vi "CaseNames To CSM States.vi"(11 "Array in":string[](array[string])) -> (3 "Array out":string[](array[string]))   [LabVIEW 2017, in "CSM-Helper.lvclass"]
uses:
  CSM-Helper.lvclass
  _Shared/CSM Shared.lvlib
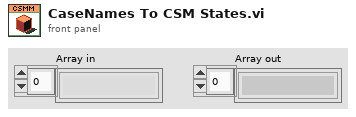
[diagram p1: front panel]
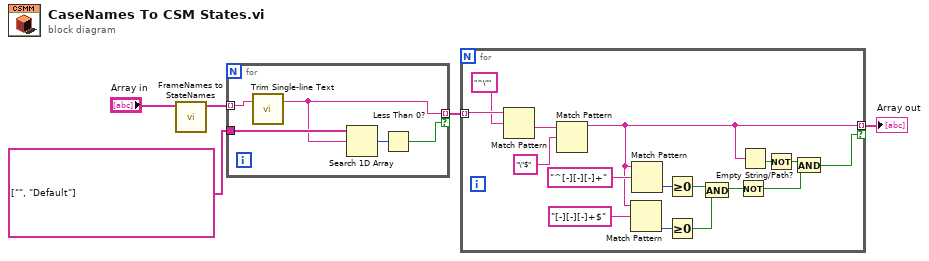
[diagram p0: block diagram]
diagram:
  n1 = call "FrameNames to StateNames.vi"("FrameNames"="Array in") -> ("Array of Strings"=w2:string[])  [unwired: 10 in]
  n2 = for {
    tunnel: w2 -> [w10] mode=indexing
    tunnel: [w8] -> w4 mode=indexing if=w6
    tunnel: string[] ["", "Default"] ("items to filter") -> [w9]
    n3 = call "Trim Single-line Text.vi"("single-line text"=w10) -> ("trimed text"=w8:string)  [unwired: 2 in]
    n4 = Search 1D Array(1D array=w9, element=w8) -> (index of element=w7:i32)  [unwired: 1 in]
    n5 = Less Than 0?(x=w7) -> (x < 0?=w6:bool)
  }
  n6 = for {
    tunnel: w4 -> [w26] mode=indexing
    tunnel: [w11] -> w5 mode=indexing if=w15
    n7 = Match Pattern(string=w26, regular expression="^\"") -> (after substring=w24:string)  [unwired: 1 in, 3 out]
    n8 = Match Pattern(string=w24, regular expression="\"$") -> (before substring=w11:string)  [unwired: 1 in, 3 out]
    n9 = Match Pattern(string=w11, regular expression="[-][-][-]+$") -> (offset past match=w19:i32)  [unwired: 1 in, 3 out]
    n10 = Match Pattern(string=w11, regular expression="^[-][-][-]+") -> (offset past match=w20:i32)  [unwired: 1 in, 3 out]
    n11 = Greater Or Equal To 0?(x=w20) -> (x >= 0?=w18:bool)
    n12 = Greater Or Equal To 0?(x=w19) -> (x >= 0?=w17:bool)
    n13 = And(x=w18, y=w17) -> (x .and. y?=w16:bool)
    n14 = Not(x=w16) -> (.not. x?=w14:bool)
    n15 = Empty String/Path?(string/path=w11) -> (empty?=w13:bool)
    n16 = Not(x=w13) -> (.not. x?=w12:bool)
    n17 = And(x=w12, y=w14) -> (x .and. y?=w15:bool)
  }
  "Array out" <- w5
